vi "Actor Core.vi"(8 "error in":errorcluster, 11 "Nested in":refnum<class "UI_Waveform.lvclass">) -> (0 "error out":errorcluster, 3 "Actor out":refnum<class "Actor.lvclass">)   [LabVIEW 2021, in "UI_Waveform.lvclass"]
doc: "(<B>Filename</B>: Actor Framework.lvlib:Actor.lvclass:Actor Core.vi)\n\nReceives messages to the actor, reacts to them, and initiates any error handling that may shut the actor down.\n\nDescendant classes may override this VI to append parallel tasks for the actor to complete while it handles messages. Overrides use the Call Parent Method node."
uses:
  UI_Waveform.lvclass
  C:/Program Files (x86)/National Instruments/LabVIEW 2021/user.lib/John_Lib/AbstractActorTemplate/AbstractActorTemplate/UIActorTop.lvclass
  C:/Program Files (x86)/National Instruments/LabVIEW 2021/vi.lib/ActorFramework/Actor/Actor.lvclass
  <vilib>/ActorFramework/Actor/Actor.lvclass
  TopRef.ctl
  UI_Waveform.lvclass/UI_Waveform.ctl
  <vilib>/ActorFramework/Actor/Actor.lvclass/Actor.ctl
  <vilib>/ActorFramework/Message Enqueuer/Message Enqueuer.lvclass/Message Enqueuer.ctl
  <vilib>/ActorFramework/Message Enqueuer/Init from Existing Queue.vi
  <vilib>/ActorFramework/Message Enqueuer/Enqueue.vi
  <vilib>/ActorFramework/Stop Msg/Stop Msg.lvclass
  C:/Program Files (x86)/National Instruments/LabVIEW 2021/vi.lib/ActorFramework/Message/Message.lvclass
  <vilib>/Utility/LVClass/Get LV Class Name.vi
  <resource>/AFDebug/Generate Trace for Message.vi
  <vilib>/ActorFramework/Message Priority Queue/Priority Enqueue.vi
  <vilib>/ActorFramework/Message Enqueuer/Message Enqueuer.lvclass
  <userlib>/John_Lib/AbstractActorTemplate/AbstractActorTemplate/UIActorTop.lvclass
panel:
  out "Waveform Graph":waveform(dbl)[](graph)
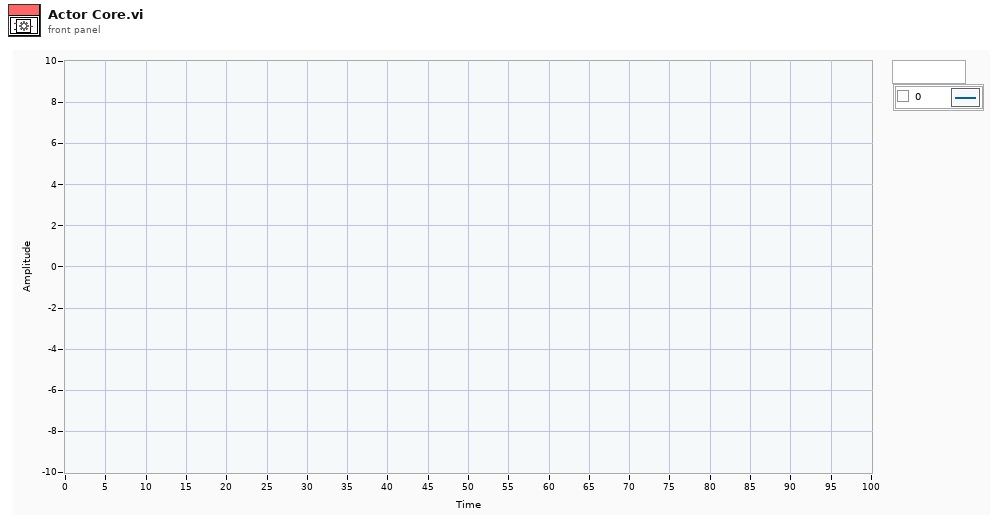
[diagram p1: front panel]
types:
  T1 = typedef "UI_Waveform.lvclass/TopRef.ctl" = cluster{"WFGraph Refnum":refnum<vi>}
  T2 = cluster{"Stop":refnum<user-event>, "Waveform Graph":refnum<user-event>}
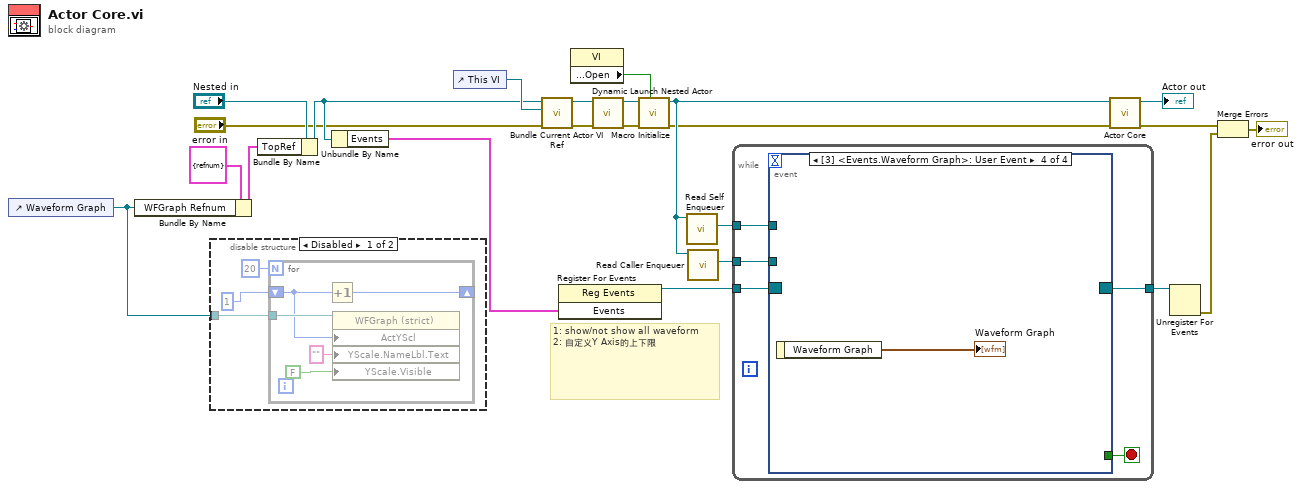
[diagram p0: block diagram]
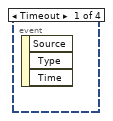
[diagram p3: hidden frame]
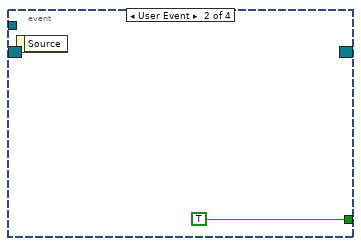
[diagram p4: hidden frame]
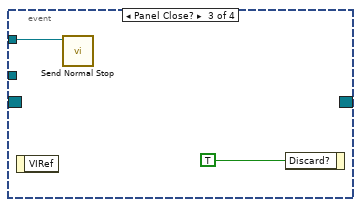
[diagram p5: hidden frame]
diagram:
  # "1: show/not show all waveform\n2: 自定义Y Axis的上下限"
  n1 = control-ref of="Waveform Graph"() -> (w2:refnum<vi>)
  n2 = Bundle By Name(cluster=T1 {"WFGraph Refnum"=refnum} ("TopRef"), "WFGraph Refnum"=w2) -> (w3:T1)
  n3 = disable-structure shown="Disabled" {
    disable-tunnel: w2 -> [w26 _]
    frame Disabled {
      n4 = for {
        N: 20 -> [_]
        tunnel: w26 -> [w31]
        shift-right: [w28] -> _
        shift-left: 1 ("Active Y Scale") -> [w29]
        n5 = Increment(x=w29) -> (x+1=w28:i32)
        n6 = property class="WFGraph (strict)"(reference=w31, "ActYScl"=w29, "YScale.NameLbl.Text"="" ("Y Scale.Name Label.Text"), "YScale.Visible"=FALSE ("Y Scale.Visible")) -> ()  [unwired: 1 in, 2 out]
      }
    }
    frame Enabled {
    }
  }
  n7 = Bundle By Name(cluster="Nested in", "TopRef"=w3) -> (w5:refnum<class "UI_Waveform.lvclass">)
  n8 = Unbundle By Name(w5) -> ("Events"=w21:T2)
  n9 = control-ref of="This VI"() -> (w6:refnum<vi>)
  n10 = call <userlib>:"Bundle Current Actor VI Ref.vi"("error in (no error)"="error in", "This VI"=w6, "UI ActorTop in"=w5) -> ("error out"=w7:errorcluster, "UI ActorTop out"=w8:refnum<class "UI_Waveform.lvclass">)  [unwired: 5 in, 2 out]
  n11 = register-events ("Main Register for Events")(w21) -> (reference out=w22:refnum<event-registration>)  [unwired: 2 in, 1 out]
  n12 = property class="VI"() -> ("Front Panel.Open"=w16:bool)  [unwired: 2 in, 2 out]
  n13 = call-dynamic "Dynamic Launch Nested Actor.vi"("error in (no error)"=w7, "UI ActorTop in"=w8) -> ("error out"=w17:errorcluster, "UI ActorTop out"=w18:refnum<class "UI_Waveform.lvclass">)  [unwired: 8 in]
  n14 = call-dynamic "Macro Initialize.vi"("Front Panel Window:Open"=w16, "error in (no error)"=w17, "UI ActorTop in"=w18) -> ("error out"=w11:errorcluster, "UI ActorTop out"=w15:refnum<class "UI_Waveform.lvclass">)  [unwired: 7 in]
  n15 = call <vilib>:"Read Self Enqueuer.vi"("Actor"=w15) -> ("Self Enqueuer"=w19:refnum<class "Message Enqueuer.lvclass">)  [unwired: 10 in]
  n16 = call <vilib>:"Read Caller Enqueuer.vi"("Actor"=w15) -> ("Caller Enqueuer"=w10:refnum<class "Message Enqueuer.lvclass">)  [unwired: 10 in]
  n17 = while {
    tunnel: w22 -> [w36]
    tunnel: [w34] -> w20
    tunnel: w19 -> [w33]
    tunnel: w10 -> [w32]
    stop <- w35 stop-if-true
    n18 = event "UI Events" shown="[3] <Events.Waveform Graph>: User Event" {
      selector: w36 -> [_ _ _ _]
      dyn-events: [_ _ _ _] -> w34
      timeout: _ -> [_ _ _ _]
      tunnel: [_ TRUE _ _] -> w35
      tunnel: w33 -> [_ _ w38 _]
      tunnel: w32 -> [_ _ _ _]
      event Timeout {
        n19 = event-data() -> ()  [unwired: 1 in, 3 out]
      }
      event User Event {
        n20 = event-data() -> ()  [unwired: 1 in, 1 out]
      }
      event Panel Close? {
        n21 = event-data() -> ()  [unwired: 1 in, 1 out]
        n22 = call <vilib>:"Send Normal Stop.vi"("Message Enqueuer"=w38) -> ()  [unwired: 10 in, 1 out]
        n23 = event-data("Discard?"=TRUE) -> ()  [unwired: 1 in, 1 out]
      }
      event User Event {
        n24 = event-data() -> ("Waveform Graph"=→"Waveform Graph":waveform(dbl)[])  [unwired: 1 in]
      }
    }
  }
  n25 = call-parent "Actor Core.vi"("error in"=w11, "Actor in"=w15) -> ("error out"=w13:errorcluster, "Actor out"=→"Actor out":refnum<class "Actor.lvclass">)  [unwired: 8 in]
  n26 = Unregister For Events(event registration refnum=w20) -> (error out=w14:errorcluster)  [unwired: 1 in]
  n27 = Merge Errors(w13, w14) -> (→"error out":errorcluster)
